vi "Set DIO Port A, B, C direction.vi"(8 "error in (no error)":errorcluster, 10 "Port A, B direction":T1, 11 "VISA resource name":refnum<visa-resource-name>) -> (0 "error out":errorcluster, 3 "VISA resource name out":refnum<visa-resource-name>)   [LabVIEW 2019, in "Newport ESP301.lvlib"]
doc: "This command is used to set digital I/O (DIO) port A and B direction where bit-0\ncorresponds to port A and B, bit-1 to port B. If any bit is set to zero(0) then its\ncorresponding port will become an input only. If any bit is set to one(1) then its\ncorresponding port will becomes an output only.\nA DIO within a port configured as an input can only report its present HIGH or\nLOW logic level. Whereas a DIO bit within a port configured as an output can\nset(1) or clear(0) the corresponding DIO hardware to HIGH or LOW logic level.\nReading the status of a port configured as output returns its present output status.\nNOTE: All direction bits are automatically zeroed, or cleared, after a system\nreset. Therefore all DIO ports default to input by default.\nNOTE: Each DIO bit has a pulled-up resistor to +5V. Therefore, all bits will be\nat HIGH logic level if not connected to external circuit and configured as input."
uses:
  Newport ESP301.lvlib
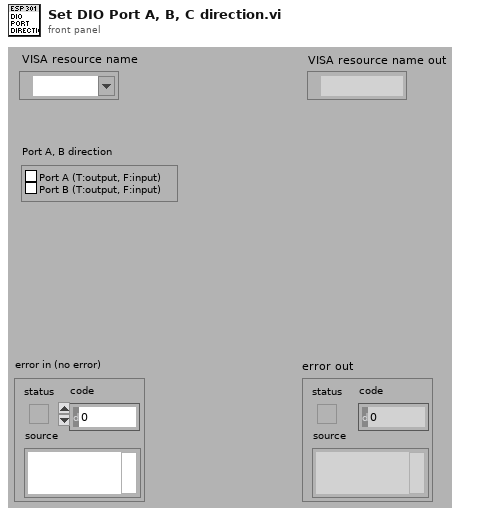
[diagram p1: front panel]
types:
  T1 = cluster{"Port A (T:output, F:input)":bool, "Port B (T:output, F:input)":bool}
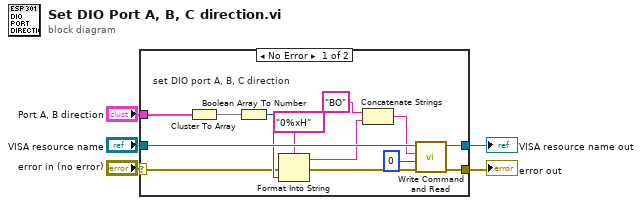
[diagram p0: block diagram]
diagram:
  n1 = case shown="No Error" "error in (no error)" {
    selector: "error in (no error)" -> [w10 w20]
    tunnel: [w17 w20] -> w5
    tunnel: "VISA resource name" -> [w18 w19]
    tunnel: [w16 w19] -> w4
    tunnel: "Port A, B direction" -> [w7 _]
    frame No Error {
      w15 = "BO"  # set DIO port A, B, C direction
      n2 = Cluster To Array(cluster=w7) -> (array=w12:bool[])
      n3 = Boolean Array To Number(Boolean array=w12) -> (number=w11:u32)
      n4 = Format Into String(format string="0%xH" ("chaîne de format"), error in=w10, w11) -> (resulting string=w8:string, error out=w9:errorcluster)  [unwired: 1 in]
      n5 = Concatenate Strings(w15, w8) -> (w14:string)
      n6 = call "Write Command and Read.vi"("error in (no error)"=w9, "Bytes to read (100)"=u32 0, "Command"=w14, "VISA resource name"=w18) -> ("error out"=w17:errorcluster, "VISA resource name out"=w16:refnum<visa-resource-name>)  [unwired: 1 in, 3 out]
    }
    frame Error {
    }
  }
  "error out" <- w5
  "VISA resource name out" <- w4
